vi "Get Strings from Ref.vi"(8 "error in (no error)":errorcluster, 9 "Label Prefix":string, 10 "GObj Refnum in":refnum<vi>, 11 "WaveformGraph in":refnum<class "IntensityChart.lvclass">) -> (0 "error out":errorcluster, 1 "Valid?":bool, 2 "GObj Refnum out":refnum<vi>, 3 "WaveformGraph out":refnum<class "IntensityChart.lvclass">, 4 "GObj Name":string)   [LabVIEW 2013, in "SET Project Data.lvlib" / "IntensityChart.lvclass"]
uses:
  IntensityChart.lvclass
  GraphChart/GraphChart.lvclass
  GObject/GObject.lvclass/GObject.ctl
  GObject/Write UID.vi
  GObject/GObject.lvclass
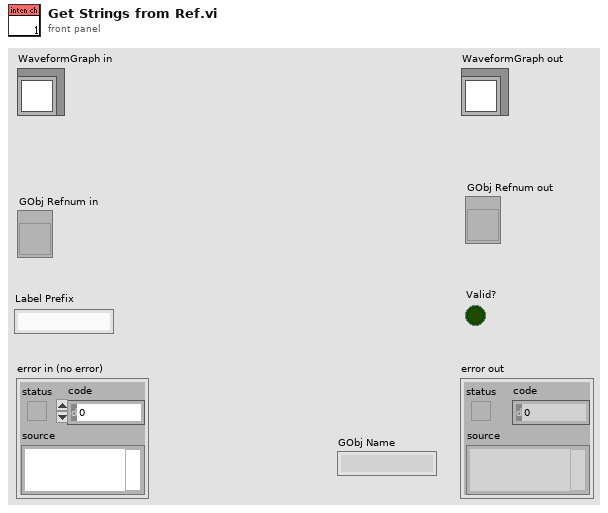
[diagram p1: front panel]
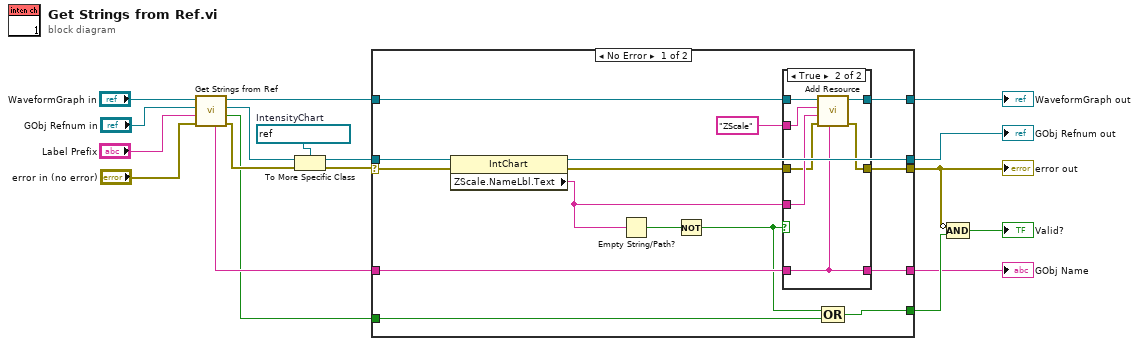
[diagram p0: block diagram]
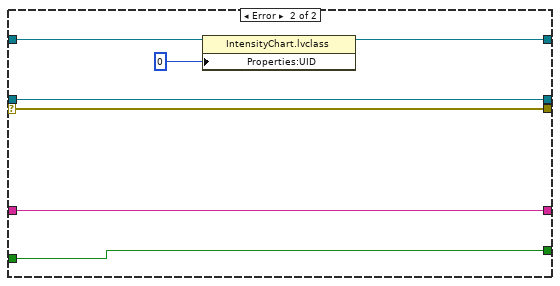
[diagram p3: hidden frame]
diagram:
  w13 = refnum<vi> refnum  # IntensityChart
  n1 = call-parent "Get Strings from Ref.vi"("error in (no error)"="error in (no error)", "Label Prefix"="Label Prefix", "GObj Refnum in"="GObj Refnum in", "GraphChart in"="WaveformGraph in") -> ("error out"=w9:errorcluster, "Valid?"=w7:bool, "GObj Refnum out"=w10:refnum<vi>, "GraphChart out"=w11:refnum<class "IntensityChart.lvclass">, "GObj Name"=w8:string)  [unwired: 3 in]
  n2 = To More Specific Class(target class=w13, reference=w10, error in=w9) -> (specific class reference=w6:refnum<vi>, error out=w12:errorcluster)
  n3 = case shown="No Error" w12 {
    selector: w12 -> [w27 w49]
    tunnel: w6 -> [w28 w50]
    tunnel: w11 -> [w33 w48]
    tunnel: [w20 w46] -> w5
    tunnel: [w22 w49] -> w2
    tunnel: [w21 w50] -> w4
    tunnel: w8 -> [w31 w45]
    tunnel: w7 -> [w30 w44]
    tunnel: [w19 w45] -> w1
    tunnel: [w29 w44] -> w14
    frame No Error {
      n4 = property class="IntChart"(reference=w28, error in=w27) -> (reference out=w21:refnum<vi>, error out=w26:errorcluster, "ZScale.NameLbl.Text"=w25:string)
      n5 = Empty String/Path?(string/path=w25) -> (empty?=w24:bool)
      n6 = Not(x=w24) -> (.not. x?=w23:bool)
      n7 = case shown="True" w23 {
        tunnel: w33 -> [w36 w43]
        tunnel: [w36 w42] -> w20
        tunnel: w31 -> [w35 w39]
        tunnel: w25 -> [_ w41]
        tunnel: "ZScale" -> [_ w40]
        tunnel: [w35 w39] -> w19
        tunnel: w26 -> [w34 w38]
        tunnel: [w34 w37] -> w22
        frame False {
        }
        frame True {
          n8 = call "Add Resource.vi"("TagPrefix"=w39, "error in (no error)"=w38, "ItemText"=w41, "ItemName"=w40, "GObject in"=w43) -> ("error out"=w37:errorcluster, "GObject out"=w42:refnum<class "IntensityChart.lvclass">)  [unwired: 5 in]
        }
      }
      n9 = Compound Arithmetic op=OR(w23, w30) -> (w29:bool)
    }
    frame Error {
      n10 = property class="IntensityChart.lvclass"(reference=w48, "Properties:UID"=0 ("UID")) -> (reference out=w46:refnum<class "IntensityChart.lvclass">)  [unwired: 1 in, 1 out]
    }
  }
  "error out" <- w2
  "WaveformGraph out" <- w5
  "GObj Refnum out" <- w4
  "GObj Name" <- w1
  n11 = Compound Arithmetic op=AND(invert w2, w14) -> (→"Valid?":bool)
